vi "Initilize Globals.vi"() -> ()   [LabVIEW 2014]
uses:
  SubVIs/ctt's/Camera Setup Acquisition.ctl
  Glimpse/Glimpse core/Image to Display event.ctt
  <vilib>/vision/Image Controls.llb/IMAQ Image.ctl
  <vilib>/Utility/miscctls.llb/LVRectTypeDef.ctl
panel:
  in  "Field mode":T1(ring)
  in  "Sequence range":cluster{i16, i16}
  in  "Stop \nAcquisition":bool
  in  "Additional error information":string
  out "Image controller display info":T3(array[cluster])
  out "Display controller Window Bounds":T4={"Left"=0, "Top"=0, "Right"=100, "Bottom"=100}
  in  "Keep mage display controller in corner?":bool=TRUE
  in  "Current window Black/White Levels":cluster{ext, ext}(slide)={1.0, 65535.0} scale=0.0..255.0
  in  "Serial Number for Image Buffers":i32
  in  "Display controller Presets":T5(array[cluster])=[{"Mem"=FALSE, "Black"=-32500.0, "White"=-25000.0, "Recall"=FALSE}]
  in  "Display image event":refnum<user-event>
  in  "Number of acquisition blocks":i8(slide)=10 scale=0.0..20.0
  in  "Pixels":cluster{"H Pixels":u32, "V Pixels":u32}
  out "Camera Acquiring":bool
  in  "Image Size":T6={"H Bin"=1.0, "V Bin"=1.0, "Left"=1.0, "Right"=1024.0, "Top"=1.0, "Bottom"=1024.0} {"V Bin" min=0.0; "H Bin" min=0.0 step=1.0}
  out "Pixel Size":dbl
  in  "Acquisition Parameters":T7={"Readout Mode"=enum."Image", "Set Acquisition Mode"=enum."Single Scan", "Trigger Mode"=enum."Internal", "Exposure Time (sec)"=1.0, "Accumulation Cycle (s)"=0.0, "Kinetic Cycle Time (s)"=1.0, "Number of Kinetics"=1, "Number of Accumulations"=1, "Set VS Speed"=1.0, "Pixel Rate"=enum."Standard CCD 3 Mhz 14 bits", "V Shift Amplitude"=enum."+1", "Preamp Gain"=enum."1.0", "Single Track Settings"={"centre"=0, "height"=1}, "EM CCD Gain"=300, "High Capacity?"=FALSE} {"EM CCD Gain" scale=0.01..300.0; "Single Track Settings"."centre" min=0 max=1024; "Single Track Settings"."height" min=1 max=1024; "Exposure Time (sec)" scale=0.001..10.0 scale format="%#_1g"; "Set VS Speed" min=0.0 format="%#_2f"}
  out "Output Amplification":i32
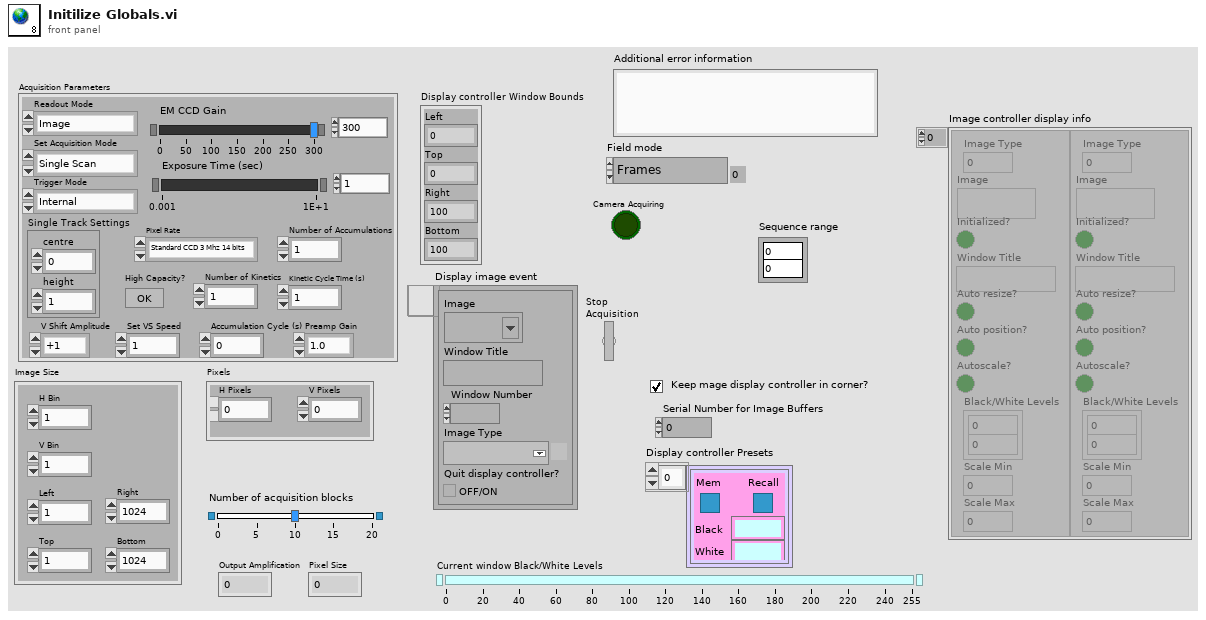
[diagram p1: front panel]
types:
  T1 = enum16{"Frames", "Fields, Odd 1st", "Fields, Even 1st", "Fields, Averaged"}
  T2 = typedef "IMAQ Image.ctl" = refnum<image>
  T3 = cluster{"Image Type":u32, "Image":T2, "Initialized?":bool, "Window Title":string, "Auto resize?":bool, "Auto position?":bool, "Autoscale?":bool, "Black/White Levels":cluster{ext, ext}, "Scale Min":ext, "Scale Max":ext}[]
  T4 = typedef "LVRectTypeDef.ctl" = cluster{"Left":i16, "Top":i16, "Right":i16, "Bottom":i16}
  T5 = cluster{"Mem":bool, "Black":ext, "White":ext, "Recall":bool}[]
  T6 = cluster{"H Bin":dbl, "V Bin":dbl, "Left":dbl, "Right":dbl, "Top":dbl, "Bottom":dbl}
  T7 = typedef "Camera Setup Acquisition.ctl" = cluster{"Readout Mode":enum16{"Full Vertical Binning", "Multi-Track", "Random-Track", "Single-Track", "Image"}, "Set Acquisition Mode":enum16{"(do nothing)", "Single Scan", "Accumulate", "Kinetics", "Fast Kinetics", "Run till abort"}, "Trigger Mode":enum16{"Internal", "External"}, "Exposure Time (sec)":sgl, "Accumulation Cycle (s)":dbl, "Kinetic Cycle Time (s)":dbl, "Number of Kinetics":i32, "Number of Accumulations":i32, "Set VS Speed":dbl, "Pixel Rate":enum16{"EM CCD 10 Mhz 14 bits", "EM CCD 5 Mhz 14 bits", "EM CCD 3 Mhz 14 bits", "EM CCD 1 Mhz 16 bits", "Standard CCD 3 Mhz 14 bits", "Standard CCD 1 Mhz 16 bits"}, "V Shift Amplitude":enum16{"normal", "+1", "+2", "+3", "+4"}, "Preamp Gain":enum16{"1.0", "2.4", "5.0"}, "Single Track Settings":cluster{"centre":i32, "height":i32}, "EM CCD Gain":u16, "High Capacity?":bool}
diagram:
